vi "AcquireWaveformsSimulated.vi"(8 "error in (no error)":errorcluster) -> (0 "error out":errorcluster, 2 "simulated pulse position array":T1[](array[typedef]), 3 "simulated waveforms":waveform(sgl)[](array[waveform]))   [LabVIEW 2017, in "CmsAcquisition.lvlib"]
uses:
  <vilib>/addons/InsightCM/Devices/Shared/Cms/CmsAcquisition/CmsAcquisition.lvlib
  <vilib>/addons/InsightCM/Utilities/Analysis/Shared/controls/PulsePositions.ctl
  <vilib>/addons/InsightCM/Utilities/Analysis/Shared/AnalysisHelper.lvlib
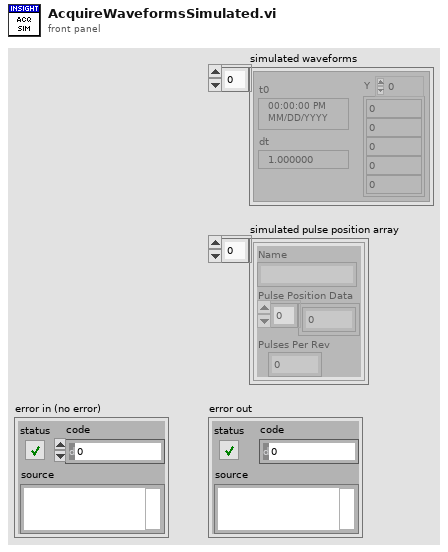
[diagram p1: front panel]
types:
  T1 = typedef "AnalysisHelper.lvlib/PulsePositions.ctl" = cluster{"Name":string, "Pulse Position Data":dbl[], "Pulses Per Rev":i32}
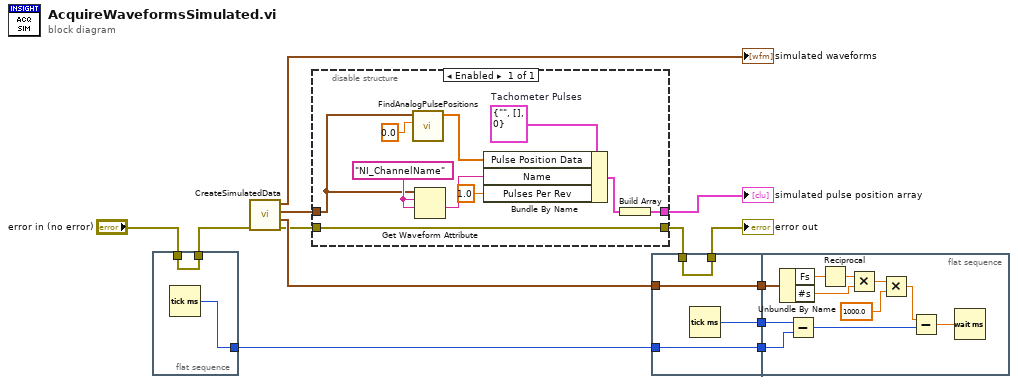
[diagram p0: block diagram]
diagram:
  n1 = flat-sequence {
    tunnel: [w15] -> w9
    tunnel: "error in (no error)" -> [w15]
    tunnel: [w14] -> w3
    frame #0 {
      n2 = Tick Count (ms)() -> (millisecond timer value=w14:u32)
    }
  }
  n3 = call <vilib>:"CreateSimulatedData.vi"("error in (no error)"=w9) -> ("error out"=w2:errorcluster, "sampling info"=w6:cluster{"Fs":dbl, "#s":dbl}, "simulated tach signal"=w12:waveform(sgl), "simulated waveforms"=→"simulated waveforms":waveform(sgl)[])  [unwired: 7 in]
  n4 = disable-structure shown="Enabled" {
    disable-tunnel: [w19] -> w13
    disable-tunnel: w12 -> [w17]
    disable-tunnel: w2 -> [w24]
    disable-tunnel: [w24] -> w1
    frame Enabled {
      w22 = T1 {"Name"="", "Pulse Position Data"=[], "Pulses Per Rev"=0}  # Tachometer Pulses
      w25 = "NI_ChannelName"
      n5 = call <vilib>:"FindAnalogPulsePositions.vi"("level"=0.0 ("Level"), "tach signal"=w17) -> ("pulse positions"=w16:dbl[])  [unwired: 9 in]
      n6 = Get Waveform Attribute(5:w25, 6:w25, 7:w17) -> (1:w20:string)  [unwired: 1 in, 3 out]
      n7 = Bundle By Name(cluster=w22, "Pulse Position Data"=w16, "Name"=w20, "Pulses Per Rev"=1.0) -> (w23:T1)
      n8 = Build Array(w23) -> (w19:T1[])
    }
  }
  "simulated pulse position array" <- w13
  n9 = flat-sequence {
    tunnel: w6 -> [w29]
    tunnel: [w29] -> w8
    tunnel: [w28] -> w7
    tunnel: [w27] -> w5
    tunnel: w1 -> [w27]
    tunnel: [w26] -> w4
    tunnel: w3 -> [w26]
    tunnel: w8 -> [w40]
    tunnel: w7 -> [w32]
    tunnel: w4 -> [w30]
    frame #0 {
      n10 = Tick Count (ms)() -> (millisecond timer value=w28:u32)
    }
    frame #1 {
      n11 = Unbundle By Name(w40) -> ("Fs"=w39:dbl, "#s"=w37:dbl)
      n12 = Subtract(x=w32, y=w30) -> (x-y=w31:u32)
      n13 = Reciprocal(x=w39) -> (1/x=w38:dbl)
      n14 = Multiply(x=w38, y=w37) -> (x*y=w36:dbl)
      n15 = Multiply(x=w36, y=1000.0) -> (x*y=w33:dbl)
      n16 = Subtract(x=w33, y=w31) -> (x-y=w34:dbl)
      n17 = Wait (ms)(milliseconds to wait=w34) -> ()  [unwired: 1 out]
    }
  }
  "error out" <- w5
